vi "TMP007 Example.vi"() -> ()   [LabVIEW 2014]
uses:
  Type Defs/tempReadings.ctl
  <vilib>/myRIO/Instrument Drivers/Onboard IO/DIO/typedefs/DIO Reference.ctl
  <vilib>/myRIO/Common/Instrument Driver Framework/Utilities/typedefs/myRIO Generic Hardware Reference.ctl
  <vilib>/myRIO/Common/Instrument Driver Framework/Utilities/typedefs/Hardware Version Enum.ctl
  <vilib>/myRIO/Common/Instrument Driver Framework/Utilities/typedefs/myRIO v1.0 Reference.ctl
  <vilib>/myRIO/Common/Instrument Driver Framework/Utilities/typedefs/Generic FPGA Reference.ctl
  <vilib>/myRIO/Common/Instrument Driver Framework/myRIO v1.0/DIO/typedefs/DIO Channels List.ctl
  <vilib>/myRIO/Common/Instrument Driver Framework/myRIO v1.0/DIO/typedefs/DIO Channels Enum.ctl
  <vilib>/userdefined/High Color/nirio_resource_hc.ctl
  <vilib>/myRIO/Common/Instrument Driver Framework/Utilities/vis/Is FPGA Ref Available.vi
  <vilib>/myRIO/Common/Instrument Driver Framework/myRIO v1.0/DIO/vis/myRIO v1.1 Open DIO.vi
  <vilib>/myRIO/Instrument Drivers/Onboard IO/DIO/vis/Write.vi
  <vilib>/myRIO/Common/Instrument Driver Framework/Utilities/vis/Validate Channels.vi
  <vilib>/myRIO/Common/Instrument Driver Framework/myRIO v1.0/DIO/vis/myRIO v1.0 Reserve DIO.vi
  <vilib>/myRIO/Common/Instrument Driver Framework/myRIO v1.0/Resource Manager/vis/myRIO v1.0 Reserve Channel List.vi
  <vilib>/myRIO/Common/Instrument Driver Framework/myRIO v1.0/DIO/vis/myRIO v1.0 Build MUX Configuration DIO.vi
  <vilib>/myRIO/Common/Instrument Driver Framework/myRIO v1.0/Resource Manager/vis/myRIO v1.0 Reserve Channel.vi
  <vilib>/myRIO/Common/Instrument Driver Framework/myRIO v1.0/Resource Manager/vis/myRIO v1.0 Unreserve Channel.vi
  <vilib>/myRIO/Common/Instrument Driver Framework/myRIO v1.0/Resource Manager/vis/myRIO v1.0 Create Configuration List.vi
  <vilib>/myRIO/Common/Instrument Driver Framework/myRIO v1.0/Resource Manager/vis/myRIO v1.0 Build Mutex Name.vi
  <vilib>/Utility/VariantDataType/GetNumericInfo.vi
  <vilib>/Utility/error.llb/Error Cluster From Error Code.vi
  <vilib>/myRIO/Common/Instrument Driver Framework/myRIO v1.0/myRIO v1.1 Open.vi
  <vilib>/myRIO/Common/Instrument Driver Framework/Utilities/vis/IO Manager.vi
  <vilib>/myRIO/Common/Instrument Driver Framework/Utilities/vis/Configuration Manager.vi
  <vilib>/myRIO/Common/Instrument Driver Framework/myRIO v1.0/Resource Manager/vis/myRIO v1.0 Configure IO.vi
  <vilib>/myRIO/Common/Instrument Driver Framework/myRIO v1.0/myRIO v1.0 Close.vi
  <vilib>/myRIO/Common/Instrument Driver Framework/myRIO v1.0/DIO/vis/myRIO v1.0 Write DIO.vi
  <vilib>/MakerHub/LINX/Public/Utilities/Open Local.vi
  <vilib>/myRIO/Express VI/Onboard IO/DO/DO Express VI.xnode
  <vilib>/myRIO/Instrument Drivers/Onboard IO/DIO/vis/myRIO DIO Open.xnode
  <vilib>/MakerHub/LINX/LMH-LINX.lvlib
  <vilib>/myRIO/Instrument Drivers/Onboard IO/DIO/DIO.lvlib
panel:
  out "Conversion Time (ms)":dbl
  out "Temp Readings":T1 {"Ambient Temp (°F)" format="%.2f °F"; "Ambient Temp (°C)" format="%.2f °C"; "Object Temp (°F)" format="%.2f °F"; "Object Temp (°C)" format="%.2f °C"}
  in  "Sensor Power (B/DIO8 (Pin 27))":bool
  in  "I2C Slave Address":u8=64 format="%x"
  in  "I2C Channel":u8
  out "Error Out":errorcluster
  out "Device Name":string
  out "ToF Loop Rate":u32
  in  "Wait (ms)":u32=10
  in  "Stop":bool
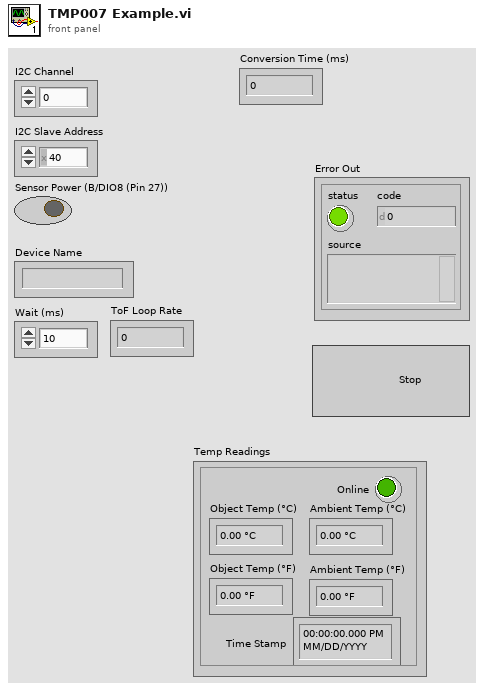
[diagram p1: front panel]
types:
  T1 = typedef "tempReadings.ctl" = cluster{"Object Temp (°C)":dbl, "Object Temp (°F)":dbl, "Ambient Temp (°C)":dbl, "Ambient Temp (°F)":dbl, "Online":bool, "Time Stamp":timestamp}
  T2 = typedef "LMH-LINX.lvlib/LINX Ref.ctl" = cluster{"IO":T3, "Interface":T4, "LINX Device Config":T5}
  T3 = typedef "LMH-LINX.lvlib/Platform.ctl" = enum16{"Remote", "Local"}
  T4 = typedef "LMH-LINX.lvlib/Interface.ctl" = enum16{"Serial", "TCP"}
  T5 = typedef "LMH-LINX.lvlib/Device.lvlib/LINX Device Config.ctl" = cluster{"Interface":T4, "COM Port":refnum<visa-resource-name>, "TCP Configuration":T6, "Device Family":u8, "Device ID":u8, "Device Name":string, "TCP Ref":refnum<k5>, "Channels":T7}
  T6 = typedef "LMH-LINX.lvlib/Device.lvlib/TCP Config.ctl" = cluster{"IP Address":string, "Port":u16}
  T7 = typedef "LMH-LINX.lvlib/Channels.ctl" = cluster{"DI":u8[], "DO":u8[], "AI":u8[], "AO":u8[], "PWM":u8[], "QE":u8[], "UART":u8[], "I2C 2":u8[], "SPI":u8[], "CAN":u8[], "Servo":u8[], "AI Ref (V)":dbl, "AI Resolution (Bits)":u8, "AO Ref (V)":dbl, "AO Resolution (Bits)":u8}
  T8 = typedef "thermopileSettings.ctl" = cluster{"Online":bool, "I2C Channel":u8, "I2C Slave Address":u8, "Valid Sample":bool, "Samples to Average":u16, "Last Temp Readings":T1, "Last Reading Time":dbl, "Last Conv Time":dbl}
  T9 = typedef "DIO.lvlib/DIO Reference.ctl" = cluster{"myRIO Reference":T10, "DIO Channels List":T14}
  T10 = typedef "myRIO Generic Hardware Reference.ctl" = cluster{"myRIO Model":T11, "myRIO Hardware Reference":T12}
  T11 = typedef "Hardware Version Enum.ctl" = enum16{"Unknown", "myRIO-1900", "myRIO-1950"}
  T12 = typedef "myRIO v1.0 Reference.ctl" = cluster{"Generic FPGA Reference":T13, "Allow multiple opens":bool}
  T13 = typedef "Generic FPGA Reference.ctl" = refnum<k20>
  T14 = typedef "DIO Channels List.ctl" = T15[]
  T15 = typedef "DIO Channels Enum.ctl" = enum16{"Not Connected", "C/DIO0", "C/DIO1", "C/DIO2", "C/DIO3", "C/DIO4", "C/DIO5", "C/DIO6", "C/DIO7", "A/DIO0", "A/DIO1", "A/DIO2", "A/DIO3", "A/DIO4", "A/DIO5", "A/DIO6", "A/DIO7", "A/DIO8", "A/DIO9", "A/DIO10", "A/DIO11", "A/DIO12", "A/DIO13", "A/DIO14", "A/DIO15", "B/DIO0", "B/DIO1", "B/DIO2", "B/DIO3", "B/DIO4", "B/DIO5", "B/DIO6", "B/DIO7", "B/DIO8", "B/DIO9", "B/DIO10", "B/DIO11", "B/DIO12", "B/DIO13", "B/DIO14", "B/DIO15", "LED0", "LED1", "LED2", "LED3", "Button0"}
  T16 = typedef "nirio_resource_hc.ctl" = tag
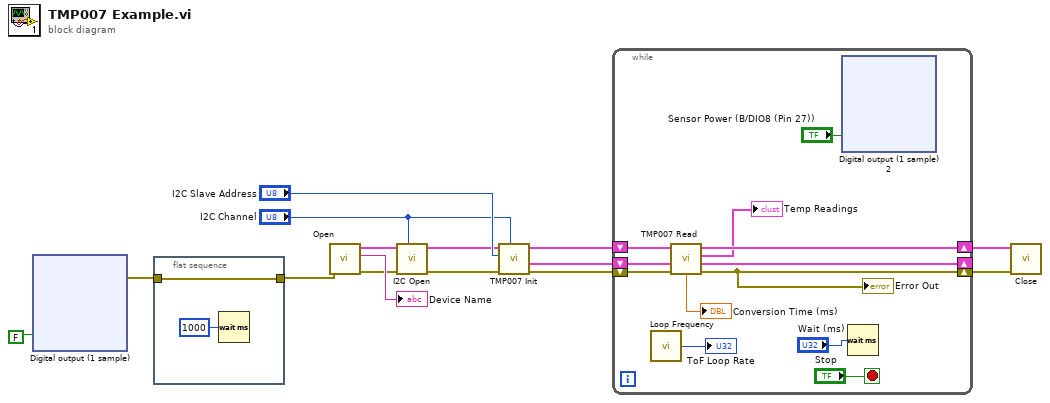
[diagram p0: block diagram]
diagram:
  n1 = xnode "Digital output (1 sample)"("Sensor Power (B/DIO8 (Pin 27))"=FALSE ("Sensor Power (B/DIO7 (Pin 25))")) -> ("error out"=w10:errorcluster)  [unwired: 1 in]
  n2 = flat-sequence {
    tunnel: w10 -> [w17]
    tunnel: [w17] -> w9
    frame #0 {
      n3 = Wait (ms)(milliseconds to wait=u32 1000) -> ()  [unwired: 1 out]
    }
  }
  n4 = call-poly <vilib>:"Open.vi"("Error In"=w9) -> ("Error Out"=w13:errorcluster, "Device Name"=→"Device Name":string, "LINX Resource"=w14:T2)  [unwired: 8 in]
  n5 = call <vilib>:"I2C Open.vi"("I2C Channel (0)"="I2C Channel", "Error In"=w13, "LINX Resource"=w14) -> ("Error Out"=w5:errorcluster, "LINX Resource"=w6:T2)  [unwired: 7 in]
  n6 = call "TMP007 Init.vi"("I2C Channel"="I2C Channel", "error in (no error)"=w5, "I2C Slave Address"="I2C Slave Address", "LINX Resource in"=w6) -> ("error out"=w4:errorcluster, "Thermopile Setting"=w1:T8, "LINX Resource out"=w3:T2)  [unwired: 5 in]
  n7 = while {
    shift-right: [w24] -> w12
    shift-left: w3 -> [w27]
    shift-right: [w23] -> w11
    shift-left: w4 -> [w26]
    shift-right: [w19] -> _
    shift-left: w1 -> [w21]
    stop <- "Stop" stop-if-true
    n8 = call <vilib>:"Loop Frequency.vi"() -> ("Loop Rate (Hz)"=→"ToF Loop Rate":u32)
    n9 = call "TMP007 Read.vi"("error in (no error)"=w26, "Thermopile Setting"=w21, "LINX Resource in"=w27) -> ("error out"=w23:errorcluster, "Thermopile Status"=w19:T8, "Temp Readings"=→"Temp Readings":T1, "LINX Resource"=w24:T2, "Conversion Time (ms)"=→"Conversion Time (ms)":dbl)  [unwired: 4 in]
    "Error Out" <- w23
    n10 = xnode "Digital output (1 sample) 2"("Sensor Power (B/DIO8 (Pin 27))"="Sensor Power (B/DIO8 (Pin 27))") -> ()  [unwired: 1 in, 1 out]
    n11 = Wait (ms)(milliseconds to wait="Wait (ms)") -> ()  [unwired: 1 out]
  }
  n12 = call <vilib>:"Close.vi"("Error In"=w11, "LINX Resource"=w12) -> ()  [unwired: 9 in, 1 out]
